vi "Compute Fit Weights.vi"(7 "Minimum Weight (1)":dbl=1.0, 9 "Use Weights? (F)":bool, 10 "Function Values":dbl[](array[numeric])) -> (2 "Weights":dbl[](array[numeric]))   [LabVIEW 2019]
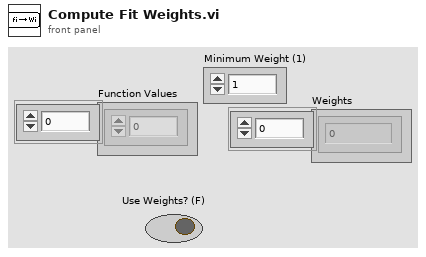
[diagram p1: front panel]
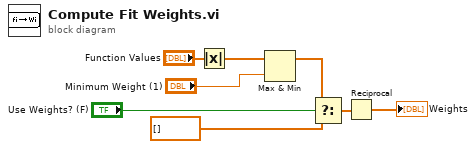
[diagram p0: block diagram]
diagram:
  n1 = Absolute Value(x="Function Values") -> (abs(x)=w5:dbl[])
  n2 = Max & Min(x=w5, y="Minimum Weight (1)") -> (max(x,y)=w1:dbl[])  [unwired: 1 out]
  n3 = Select(t=w1, s="Use Weights? (F)", f=dbl[] []) -> (s? t:f=w6:dbl[])
  n4 = Reciprocal(x=w6) -> (1/x=→"Weights":dbl[])
